vi "Vision Processing.vi"(4 "error in (no error)":errorcluster, 6 "CameraDevRef":T1) -> ()   [LabVIEW 2011]
uses:
  <vilib>/Rock Robotics/WPI/Camera/WPI_CameraDevRef.ctl
  Robot Global Data.vi
  <vilib>/vision/NI_Vision_Development_Module.lvlib
panel:
  in  "AntiDrift":dbl
  in  "Y AbsolVal Difference":dbl=0.25
  in  "Default Shooter Speed Dump":dbl=0.4
  in  "Scale":dbl=0.85
  in  "Minimum Power":dbl=0.22
  out "Aspect Ratio":dbl[](array[numeric])
  out "Offset":dbl
  out "Raw Turret":dbl
  out "Target X Coord":dbl
  out "Target Distance":dbl
  out "Distance Array":dbl[](array[numeric])
  in  "Dead Band":dbl=0.09
  out "Number of Rectangles Visible":dbl
  out "Y Position Array":dbl[](array[numeric])
  out "X Position Array":dbl[](array[numeric])
  in  "View":bool
  out "Target Info":T2(array[cluster])
  in  "Area Size Limit":i32=444
  in  "Particle Count Limit":i32=8
  in  "Score Limits":T3={"Rect Coverage"=76.0, "Aspect Ratio"=40.0, "X Edge Strength"=40.0, "Y Edge Strength"=60.0}
  in  "Processing":enum32{"Color", "Intensity", "Intensity Open"}(tab)=enum."Intensity"
  in  "Luminance":i32=255
  in  "Saturation":i32=255
  in  "Hue":i32(knob)=65 scale=0.0..255.0
  in  "Margins":cluster{"Hue":i32, "Sat":i32, "Lum":i32}={"Hue"=20, "Sat"=27, "Lum"=30} {"Sat" scale=0.0..40.0; "Lum" scale=0.0..40.0; "Hue" scale=0.0..40.0}
  in  "Range":cluster{"Lower value":sgl, "Upper value":sgl}={"Lower value"=151.52174, "Upper value"=255.0} {"Lower value" scale=0.0..255.0; "Upper value" scale=0.0..255.0}
  in  "Range":cluster{"Lower value":sgl, "Upper value":sgl}={"Lower value"=123.804344, "Upper value"=255.0} {"Lower value" scale=0.0..255.0; "Upper value" scale=0.0..255.0}
  in  "View":bool
  out "Processed Image":T4(plugin-control)
  out "Original Image":T4(plugin-control)
  # "Instructions:\nProcessing the reflective tape that is illuminated by a ring light can be based\non color or light intensity.\nParticles within the image are scored by rectangle coverage, aspect ratio, and\nfor being hollow with a bold edge. A particle is considered a target if all scores\nare above the score limits. Particles can be annotated -- surrounded by\na rectangle and scores drawn to the left .\nTo control the number of particles being scored, use the count limit and the size\nlimit."
  # "-0.065"
  # "(in)"
  # "To debug, Enable using the View button.\nFor color processing, you can click in the image to select the color for processing."
  # "Enable by clicking the View button.\nGreen scores are above the limit, orange are below. Inner/outer rect\nindicates all passed."
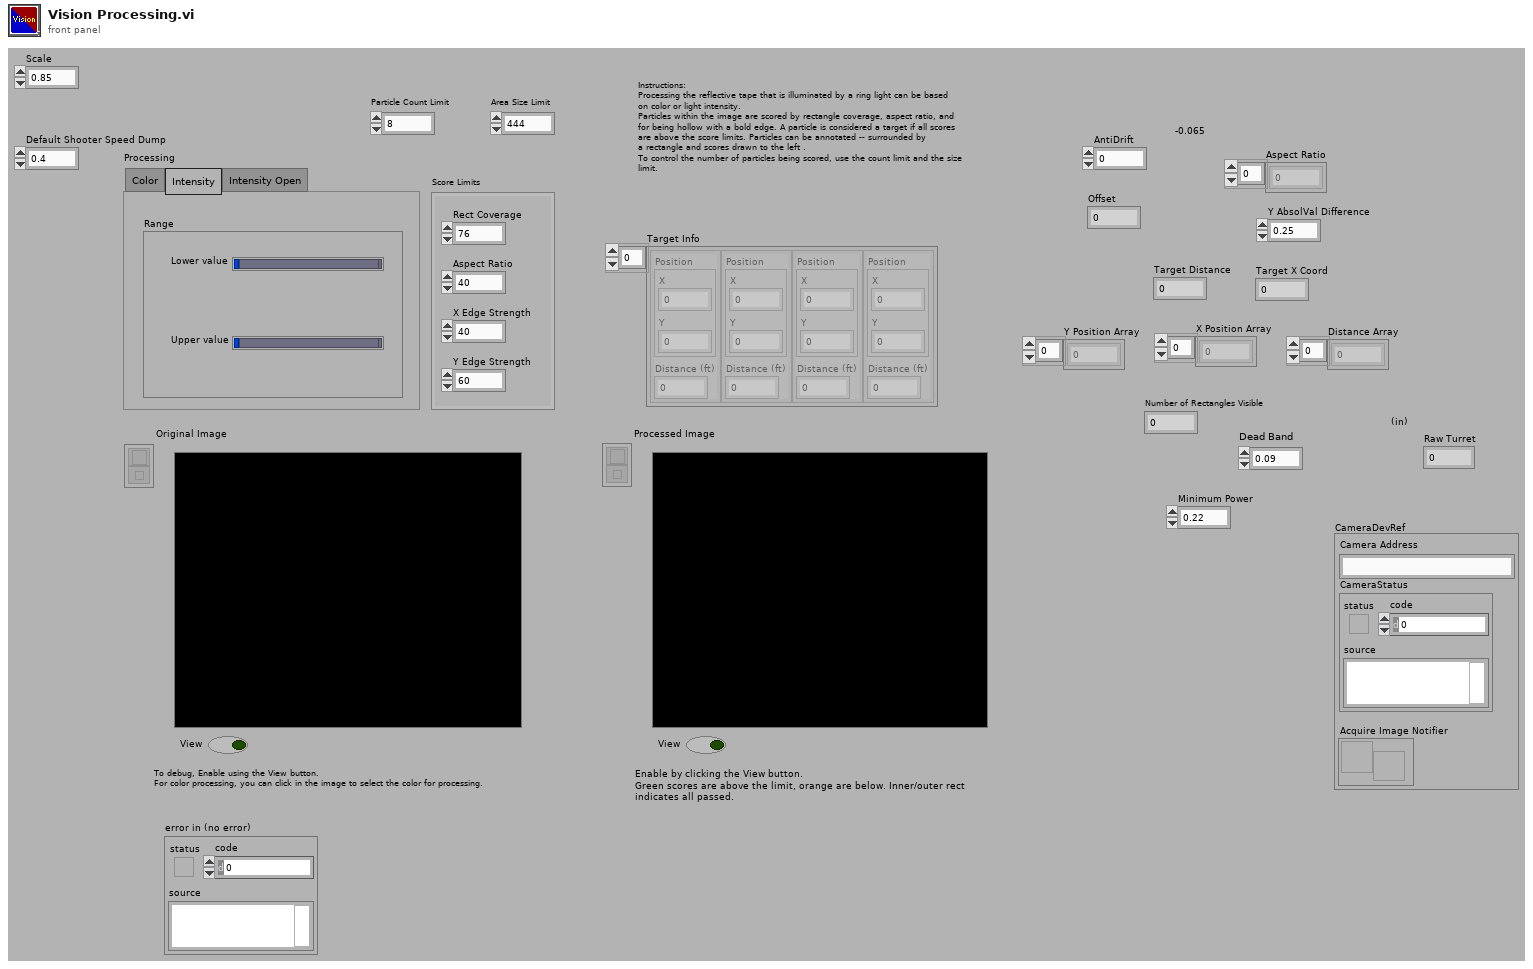
[diagram p1: front panel]
types:
  T1 = typedef "WPI_CameraDevRef.ctl" = cluster{"Camera Address":string, "CameraStatus":errorcluster, "Acquire Image Notifier":refnum<notifier>}
  T2 = cluster{"Position":cluster{"X":dbl, "Y":dbl}, "Distance (ft)":dbl}[]
  T3 = cluster{"Rect Coverage":dbl, "Aspect Ratio":dbl, "X Edge Strength":dbl, "Y Edge Strength":dbl}
  T4 = typedef "IMAQ Image.ctl" = refnum<image>
  T5 = typedef "Image Type" = u32
  T6 = enum32{"AutoM", "Close", "Dilate", "Erode", "Gradient", "Gradient out", "Gradient in", "Hit miss", "Open", "PClose", "POpen", "Thick", "Thin"}
  T7 = typedef "WPI_CameraImageSize.ctl" = enum16{"640x480", "320x240", "160x120"}
  T8 = cluster{"fps":i32, "compression":i32, "Image Size":T7}
  T9 = cluster{cluster{"Left":dbl, "Top":dbl, "Right":dbl, "Bottom":dbl}, dbl[]}[]
  T10 = cluster{"Left":dbl, "Top":dbl, "Right":dbl, "Bottom":dbl}
  T11 = cluster{"Target Center (-1 to 1)":cluster{"X":dbl, "Y":dbl}, "Distance (ft)":dbl}
  T12 = cluster{"Target Center (-1 to 1)":cluster{"X":dbl, "Y":dbl}, "Distance (ft)":dbl}[]
  T13 = typedef "WPI_JoystickDevRef.ctl" = cluster{"Device":T14}
  T14 = typedef "WPI_JoystickDeviceEnum.ctl" = enum16{"USB 1", "USB 2", "USB 3", "USB 4", "Kinect 1", "Kinect 2"}
  T15 = typedef "WPI_JoystickButtonState.ctl" = cluster{"Button 1":bool, "Button 2":bool, "Button 3":bool, "Button 4":bool, "Button 5":bool, "Button 6":bool, "Button 7":bool, "Button 8":bool, "Button 9":bool, "Button 10":bool, "Button 11":bool, "Button 12":bool}
  T16 = cluster{"axis 1 (x)":dbl, "axis 2 (y)":dbl, "axis 3 (throttle)":dbl, "axis 4":dbl, "axis 5":dbl, "axis 6":dbl}
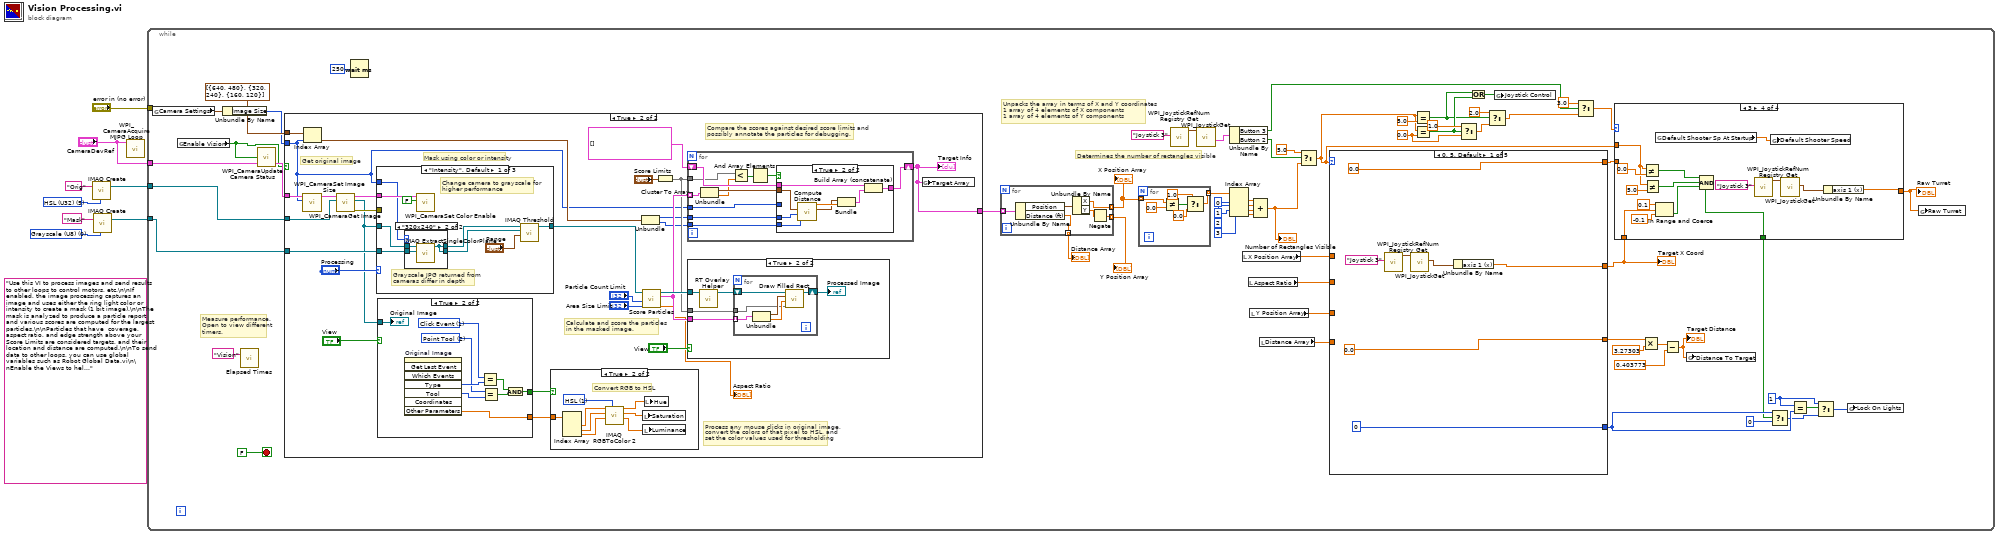
[diagram p0: block diagram]
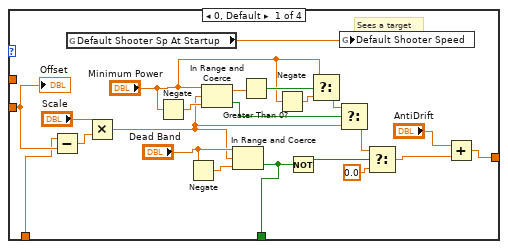
[diagram p2: hidden frame]
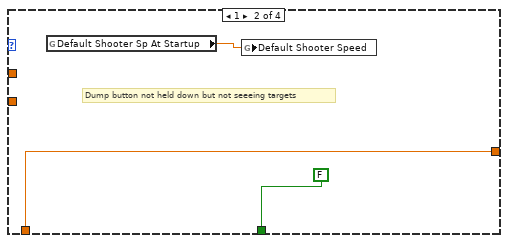
[diagram p3: hidden frame]
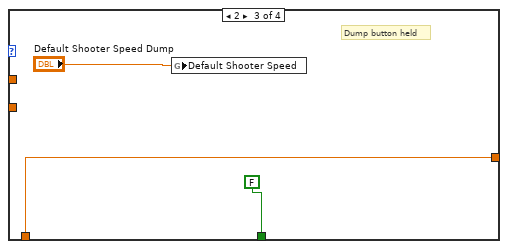
[diagram p4: hidden frame]
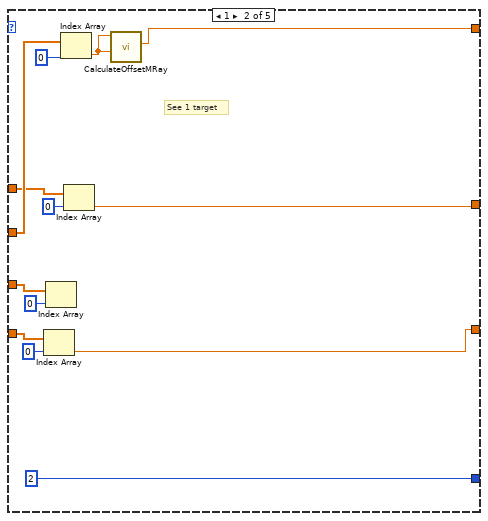
[diagram p5: hidden frame]
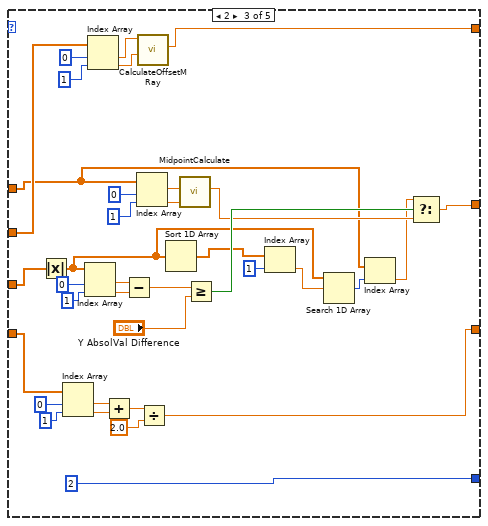
[diagram p6: hidden frame]
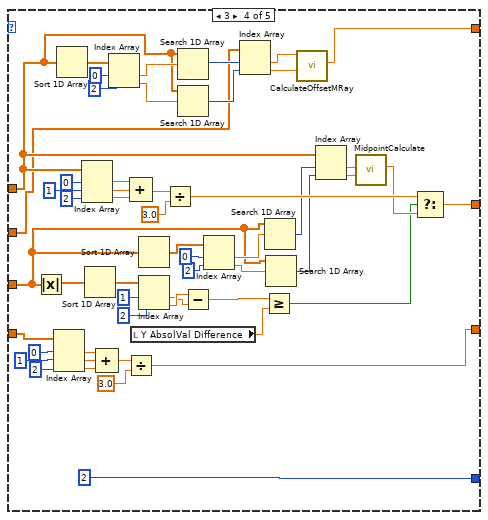
[diagram p7: hidden frame]
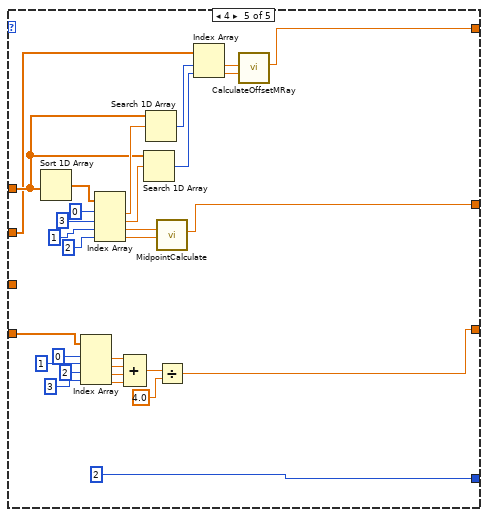
[diagram p8: hidden frame]
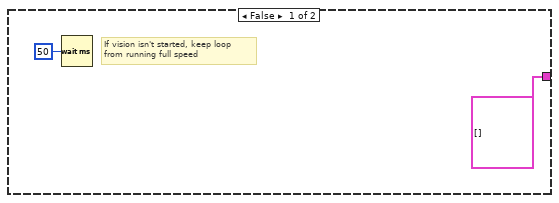
[diagram p9: hidden frame]
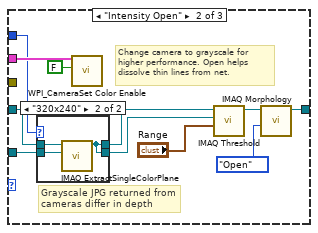
[diagram p12: hidden frame]
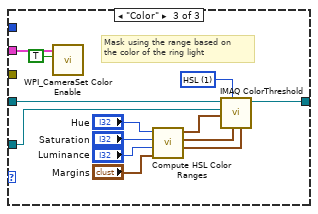
[diagram p14: hidden frame]
diagram:
  w3 = T5 0 items=["Grayscale (U8)", "Grayscale (I16)", "Grayscale (SGL)", "Complex (CSG)", "RGB (U32)", "HSL (U32)", "RGB (U64)", "Grayscale (U16)"] ("Image Type")
  (unwired) "Use this VI to process images and send results to other loops to control motors, etc.\n\nIf enabled, the image processing captures an image and uses either the ring light color or intensity to create a mask (1 bit image).\n\nThe mask is analyzed to produce a particle report and various scores are computed for the largest particles.\n\nParticles that have  coverage, aspect ratio, and edge strength above your Score Limits are considered targets, and their location and distance are computed.\n\nTo send data to other loops, you can use global variables such as Robot Global Data.vi\n\nEnable the Views to help debug color settings. Disable the View to speed up processing."
  w7 = T5 5 items=["Grayscale (U8)", "Grayscale (I16)", "Grayscale (SGL)", "Complex (CSG)", "RGB (U32)", "HSL (U32)", "RGB (U64)", "Grayscale (U16)"] ("Image Type")
  n1 = call "IMAQ Create"("Image Name"="Orig", "Image Type"=w7) -> ("New Image"=w6:T4)  [unwired: 2 in, 2 out]
  n2 = call "IMAQ Create"("Image Name"="Mask", "Image Type"=w3) -> ("New Image"=w1:T4)  [unwired: 2 in, 2 out]
  n3 = call <vilib>:"WPI_CameraAcquire MJPG Loop.vi"("CameraDevRef"="CameraDevRef") -> ()  [unwired: 11 in]
  n4 = while {
    tunnel: w6 -> [w69]
    tunnel: "CameraDevRef" -> [w68]
    tunnel: "error in (no error)" -> [_]
    tunnel: w1 -> [w64]
    stop <- FALSE stop-if-true
    w17 = 0.0 ("y")
    w34 = 1 ("y")
    # "Determines the number of rectangles visible"
    # "Unpacks the array in terms of X and Y coordinates\n1 array of 4 elements of X components\n1 array of 4 elements of Y components"
    # "Measure performance.\nOpen to view different\ntimers."
    n5 = global read "Robot Global Data.vi" "Camera Settings"() -> (w62:T8)
    n6 = global read "Robot Global Data.vi" "Enable Vision"() -> (w66:bool)
    n7 = Unbundle By Name(w62) -> ("Image Size"=w61:T7)
    n8 = call "Elapsed Times.vi"("Call Name"="Vision") -> ()  [unwired: 2 in, 1 out]
    n9 = call <vilib>:"WPI_CameraUpdate Camera Status.vi"("CameraDevRef In"=w68, "Enable Vision"=w66) -> ("CameraDevRef Out"=w67:T1)  [unwired: 3 in]
    n10 = case shown="True" w66 {
      tunnel: w69 -> [_ w284]
      tunnel: w67 -> [_ w280]
      tunnel: w64 -> [_ w271]
      tunnel: cluster{i32, i32}[] [{640, 480}, {320, 240}, {160, 120}] -> [_ w275]
      tunnel: w61 -> [_ w268]
      tunnel: [T2 [] w269] -> w60
      frame False {
        # "If vision isn't started, keep loop\nfrom running full speed"
        n11 = Wait (ms)(milliseconds to wait=u32 50) -> ()  [unwired: 1 out]
      }
      frame True {
        # "Compare the scores against desired score limits and\npossibly annotate the particles for debugging."
        # "Process any mouse clicks in original image,\nconvert the colors of that pixel to HSL, and\nset the color values used for thresholding"
        # "Calculate and score the particles\nin the masked image."
        # "Mask using color or intensity"
        # "Get original image"
        n12 = call <vilib>:"WPI_CameraSet Image Size.vi"("Image Size"=w268, "CameraDevRef"=w280) -> ("CameraDevRef Out"=w281:T1)  [unwired: 8 in, 1 out]
        n13 = Index Array(array=w275, index=w268) -> (element=w272:cluster{i32, i32})
        n14 = call <vilib>:"WPI_CameraGet Image.vi"("Image"=w284, "CameraDevRef"=w281) -> ("error out"=w282:errorcluster, "Image Out"=w270:T4, "CameraDevRef Out"=w283:T1)  [unwired: 7 in]
        n15 = case shown="\"Intensity\", Default" "Processing" {
          tunnel: w270 -> [w306 w318 w344]
          tunnel: [w309 w323 w343] -> w278
          tunnel: w283 -> [w307 w321 w334]
          tunnel: w282 -> [_ _ _]
          tunnel: w271 -> [w305 w319 w332]
          tunnel: w268 -> [w304 w320 _]
          frame "Intensity", Default {
            # "Grayscale JPG returned from\ncameras differ in depth"
            # "Change camera to grayscale for\nhigher performance"
            n16 = case shown="\"320x240\"" w304 {
              tunnel: w306 -> [w312 w315]
              tunnel: w305 -> [w311 w314]
              tunnel: [w312 w313] -> w303
              tunnel: [w311 w313] -> w302
              frame "640x480", Default {
              }
              frame "320x240" {
                n17 = call "IMAQ ExtractSingleColorPlane"("Image Dst"=w314, "Image Src"=w315) -> ("Image Dst Out"=w313:T4)  [unwired: 8 in, 1 out]
              }
            }
            n18 = call <vilib>:"WPI_CameraSet Color Enable.vi"("Color Enabled"=FALSE, "CameraDevRef"=w307) -> ()  [unwired: 8 in, 2 out]
            n19 = call "IMAQ Threshold"("Range"="Range", "Image Dst"=w302, "Image Src"=w303) -> ("Image Dst Out"=w309:T4)  [unwired: 3 in, 5 out]
          }
          frame "Intensity Open" {
            # "Grayscale JPG returned from\ncameras differ in depth"
            # "Change camera to grayscale for\nhigher performance. Open helps\ndissolve thin lines from net."
            n20 = case shown="\"320x240\"" w320 {
              tunnel: w318 -> [w328 w331]
              tunnel: w319 -> [w327 w330]
              tunnel: [w328 w329] -> w317
              tunnel: [w327 w329] -> w316
              frame "640x480", Default {
              }
              frame "320x240" {
                n21 = call "IMAQ ExtractSingleColorPlane"("Image Dst"=w330, "Image Src"=w331) -> ("Image Dst Out"=w329:T4)  [unwired: 8 in, 1 out]
              }
            }
            n22 = call <vilib>:"WPI_CameraSet Color Enable.vi"("Color Enabled"=FALSE, "CameraDevRef"=w321) -> ()  [unwired: 8 in, 2 out]
            n23 = call "IMAQ Threshold"("Range"="Range", "Image Dst"=w316, "Image Src"=w317) -> ("Image Dst Out"=w324:T4)  [unwired: 3 in, 5 out]
            n24 = call "IMAQ Morphology"("Operation"=T6."Open", "Image Src"=w324) -> ("Image Dst Out"=w323:T4)  [unwired: 8 in, 1 out]
          }
          frame "Color" {
            w342 = u16 1 items=["RGB", "HSL", "HSV", "HSI"] ("Color Mode")
            # "Mask using the range based on\nthe color of the ring light"
            n25 = call <vilib>:"WPI_CameraSet Color Enable.vi"("Color Enabled"=TRUE, "CameraDevRef"=w334) -> ()  [unwired: 8 in, 2 out]
            n26 = call "Compute HSL Color Ranges.vi"("Margins"="Margins", "Luminance"="Luminance", "Saturation"="Saturation", "Hue"="Hue") -> ("Lum Range"=w339:cluster{i32, i32}, "Sat Range"=w340:cluster{i32, i32}, "Hue Range"=w341:cluster{i32, i32})  [unwired: 5 in]
            n27 = call "IMAQ ColorThreshold"("Blue or Luma or Val or Inten Range"=w339, "Green or Sat Range"=w340, "Color Mode"=w342, "Red or Hue Range"=w341, "Image Dst"=w332, "Image Src"=w344) -> ("Image Dst Out"=w343:T4)  [unwired: 4 in, 1 out]
          }
        }
        n28 = case shown="True" "View" {
          tunnel: w270 -> [_ w364]
          tunnel: [_ w359] -> w277
          tunnel: [_ w356] -> w276
          frame False {
          }
          frame True {
            w357 = 2 items=["None", "Selection Tool", "Point Tool", "Line Tool", "Rectangle Tool", "Oval Tool", "Polygon Tool", "ClosedFreehandTool", "Annulus Tool", "Rotated Rectangle Tool", "Zoom Tool", "Pan Tool", "Polyline Tool", "Freehand Tool"] ("Tool")
            w358 = 1 items=["No Event"=0, "Click Event"=1, "Draw Event"=2, "Size Event"=4, "Scroll Event"=5, "Double Click Event"=8] ("Type")
            n29 = invoke on="Original Image" class="ImageControl" method="Get Last Event"() -> ("Type"=w360:i32, "Tool"=w363:i32, "Other Parameters"=w356:sgl[])  [unwired: 8 in, 5 out]
            n30 = Equal?(x=w358, y=w360) -> (x = y?=w361:bool)
            n31 = Equal?(x=w357, y=w363) -> (x = y?=w362:bool)
            n32 = And(x=w361, y=w362) -> (x .and. y?=w359:bool)
            "Original Image" <- w364
          }
        }
        n33 = case shown="True" w277 {
          tunnel: w276 -> [_ w301]
          frame False {
          }
          frame True {
            w300 = u16 1 items=["RGB", "HSL", "HSV", "HSI", "CIE L*a*b*", "CIE XYZ"] ("Color Mode")
            # "Convert RGB to HSL"
            n34 = Index Array(array=w301) -> (element #1=w299:sgl, element #2=w297:sgl, element #3=w295:sgl)  [unwired: 3 in]
            n35 = call "IMAQ RGBToColor 2"("Color Mode"=w300, "Blue value"=w295, "Green value"=w297, "Red value"=w299) -> ("Blue or Luma or Val or Inten or Z or b*value"=w294:dbl, "Green or Sat or Y or a* value"=w296:dbl, "Red or Hue or X or L* value"=w298:dbl)  [unwired: 4 in, 1 out]
            n36 = local write "Saturation"(w296) -> ()
            n37 = local write "Luminance"(w294) -> ()
            n38 = local write "Hue"(w298) -> ()
          }
        }
        n39 = Unbundle(w272) -> (w274:i32, w273:i32)
        n40 = call "Score Particles.vi"("Area Size Limit"="Area Size Limit", "Particle Count Limit"="Particle Count Limit", "Image Refnum in"=w278) -> ("Aspect Ratio"=→"Aspect Ratio":dbl[], "Scored Particle Info"=w289:T9, "Image Refnum out"=w292:T4)  [unwired: 6 in]
        n41 = Cluster To Array(cluster="Score Limits") -> (array=w287:dbl[])
        n42 = for {
          shift-right: [w374] -> w269
          shift-left: T2 [] -> [w375]
          tunnel: w274 -> [w373]
          tunnel: w289 -> [w371] mode=indexing
          tunnel: w287 -> [w366]
          tunnel: w268 -> [w370]
          tunnel: w273 -> [w365]
          n43 = Unbundle(w371) -> (w372:T10, w367:dbl[])
          n44 = Less?(x=w366, y=w367) -> (x < y?=w369:bool[])
          n45 = And Array Elements(Boolean array=w369) -> (logical AND=w368:bool)
          n46 = case shown="True" w368 {
            tunnel: w375 -> [w376 w384]
            tunnel: [w376 w383] -> w374
            tunnel: w372 -> [_ w379]
            tunnel: w373 -> [_ w381]
            tunnel: w370 -> [_ _]
            tunnel: w365 -> [_ w378]
            frame False {
            }
            frame True {
              n47 = call "Compute Distance.vi"("Y Image Resolution"=w378, "X Image Resolution"=w381, "Bounding Box"=w379) -> ("Target Center (-1 to 1)"=w377:cluster{"X":dbl, "Y":dbl}, "Distance (ft)"=w380:dbl)  [unwired: 7 in]
              n48 = Bundle("Target Center (-1 to 1)"=w377, "Distance (ft)"=w380) -> (w382:T11)  [unwired: 1 in]
              n49 = Build Array (concatenate)(w384, w382) -> (w383:T12)
            }
          }
        }
        "Target Info" <- w269
        n50 = case shown="True" "View" {
          tunnel: w292 -> [_ w346]
          tunnel: w289 -> [_ w348]
          tunnel: w287 -> [_ w347]
          frame False {
          }
          frame True {
            n51 = call "RT Overlay Helper.vi"("Refnum in"=w346) -> ("Refnum out"=w349:T4)  [unwired: 10 in]
            n52 = for {
              shift-right: [w354] -> w345
              shift-left: w349 -> [w355]
              tunnel: w348 -> [w351] mode=indexing
              tunnel: w347 -> [w350]
              n53 = Unbundle(w351) -> (w352:T10, w353:dbl[])
              n54 = call "Draw Filled Rect.vi"("Limits"=w350, "Scores"=w353, "Bounding Box"=w352, "image in"=w355) -> ("image out"=w354:T4)  [unwired: 7 in]
            }
            "Processed Image" <- w345
          }
        }
        n55 = global write "Robot Global Data.vi" "Target Array"(w269) -> ()
      }
    }
    n56 = Wait (ms)(milliseconds to wait=u32 250) -> ()  [unwired: 1 out]
    n57 = for {
      tunnel: [w262] -> w40 mode=indexing
      tunnel: [w263] -> w50 mode=indexing
      tunnel: w60 -> [w260] mode=indexing
      tunnel: [w259] -> w52 mode=indexing
      n58 = Unbundle By Name(w260) -> ("Position"=w264:cluster{"X":dbl, "Y":dbl}, "Distance (ft)"=w259:dbl)
      n59 = Unbundle By Name(w264) -> ("X"=w263:dbl, "Y"=w261:dbl)
      n60 = Negate(x=w261) -> (-x=w262:dbl)
    }
    "X Position Array" <- w50
    "Y Position Array" <- w40
    "Distance Array" <- w52
    n61 = for {
      tunnel: w50 -> [w118] mode=indexing
      tunnel: [w114] -> w49 mode=indexing
      n62 = Not Equal?(x=w118, y=0.0) -> (x != y?=w117:bool)
      n63 = Select(t=1.0, s=w117, f=0.0) -> (s? t:f=w114:dbl)
    }
    n64 = call <vilib>:"WPI_JoystickRefNum Registry Get.vi"("refnum name"="Joystick 3") -> ("JoystickDevRef"=w39:T13)  [unwired: 9 in, 1 out]
    n65 = call <vilib>:"WPI_JoystickGet.vi"("JoystickDevRef"=w39) -> ("Buttons"=w37:T15)  [unwired: 4 in, 2 out]
    n66 = Unbundle By Name(w37) -> ("Button 3"=w11:bool, "Button 2"=w36:bool)
    n67 = Index Array(array=w49, index #1=0 ("index"), index #2=1 ("index"), index #3=2 ("index"), index #4=3 ("index")) -> (element #1=w47:dbl, element #2=w48:dbl, element #3=w46:dbl, element #4=w45:dbl)
    n68 = local read "X Position Array"() -> (w51:dbl[])
    n69 = local read "Aspect Ratio"() -> (w29:dbl[])
    n70 = local read "Y Position Array"() -> (w53:dbl[])
    n71 = Compound Arithmetic op=ADD(w47, w48, w46, w45) -> (w30:dbl)
    "Number of Rectangles Visible" <- w30
    n72 = local read "Distance Array"() -> (w54:dbl[])
    n73 = Select(t=5.0, s=w36, f=w30) -> (s? t:f=w9:dbl)
    n74 = case shown="0, 5, Default" w9 {
      tunnel: w51 -> [_ w134 w141 w183 w234]
      tunnel: [w122 w133 w165 w217 w257] -> w27
      tunnel: w53 -> [_ w131 w164 w195 _]
      tunnel: w54 -> [_ w129 w153 w226 w254]
      tunnel: [0 2 2 2 2] -> w33
      tunnel: [0.0 ("Offset") w136 w170 w176 w243] -> w28
      tunnel: w29 -> [_ w139 w173 w179 w229]
      tunnel: [0.0 w128 w148 w219 w244] -> w22
      frame 0, 5, Default {
        n75 = call <vilib>:"WPI_JoystickRefNum Registry Get.vi"("refnum name"="Joystick 3") -> ("JoystickDevRef"=w121:T13)  [unwired: 9 in, 1 out]
        n76 = call <vilib>:"WPI_JoystickGet.vi"("JoystickDevRef"=w121) -> ("Axes"=w123:T16)  [unwired: 4 in, 2 out]
        n77 = Unbundle By Name(w123) -> ("axis 1 (x)"=w122:dbl)
      }
      frame 1 {
        # "See 1 target"
        n78 = Index Array(array=w129, index=0) -> (element=w128:dbl)
        n79 = Index Array(array=w131, index=0) -> ()  [unwired: 1 out]
        n80 = Index Array(array=w139, index=0) -> (element=w137:dbl)
        n81 = Index Array(array=w134, index=0) -> (element=w133:dbl)
        n82 = call "CalculateOffsetMRay.vi"("AR2"=w137, "AR1"=w137) -> ("Offset"=w136:dbl)  [unwired: 9 in]
      }
      frame 2 {
        n83 = Absolute Value(x=w164) -> (abs(x)=w144:dbl[])
        n84 = Index Array(array=w153, index #1=0 ("index"), index #2=1 ("index")) -> (element #1=w151:dbl, element #2=w152:dbl)
        n85 = Index Array(array=w144, index #1=0 ("index"), index #2=1 ("index")) -> (element #1=w160:dbl, element #2=w161:dbl)
        n86 = Index Array(array=w173, index #1=0 ("index"), index #2=1 ("index")) -> (element #1=w172:dbl, element #2=w171:dbl)
        n87 = Add(x=w151, y=w152) -> (x+y=w150:dbl)
        n88 = Subtract(x=w160, y=w161) -> (x-y=w159:dbl)
        n89 = Index Array(array=w141, index #1=0 ("index"), index #2=1 ("index")) -> (element #1=w166:dbl, element #2=w167:dbl)
        n90 = call "CalculateOffsetMRay.vi"("AR2"=w171, "AR1"=w172) -> ("Offset"=w170:dbl)  [unwired: 9 in]
        n91 = Divide(x=w150, y=2.0) -> (x/y=w148:dbl)
        n92 = Sort 1D Array(array=w144) -> (sorted array=w146:dbl[])
        n93 = call "MidpointCalculate.vi"("X2"=w167, "X1"=w166) -> ("Midpoint"=w156:dbl)  [unwired: 9 in]
        n94 = Greater Or Equal?(x=w159, y="Y AbsolVal Difference") -> (x >= y?=w157:bool)
        n95 = Index Array(array=w146, index=1) -> (element=w143:dbl)
        n96 = Search 1D Array(1D array=w144, element=w143) -> (index of element=w142:i32)  [unwired: 1 in]
        n97 = Index Array(array=w141, index=w142) -> (element=w140:dbl)
        n98 = Select(t=w140, s=w157, f=w156) -> (s? t:f=w165:dbl)
      }
      frame 3 {
        n99 = Absolute Value(x=w195) -> (abs(x)=w216:dbl[])
        n100 = Index Array(array=w226, index #1=0 ("index"), index #2=1 ("index"), index #3=2 ("index")) -> (element #1=w222:dbl, element #2=w223:dbl, element #3=w224:dbl)
        n101 = Sort 1D Array(array=w183) -> (sorted array=w187:dbl[])
        n102 = Index Array(array=w183, index #1=0 ("index"), index #2=1 ("index"), index #3=2 ("index")) -> (element #1=w204:dbl, element #2=w206:dbl, element #3=w205:dbl)
        n103 = Sort 1D Array(array=w216) -> (sorted array=w200:dbl[])
        n104 = Compound Arithmetic op=ADD(w222, w223, w224) -> (w221:dbl)
        n105 = Index Array(array=w187, index #1=0 ("index"), index #2=2 ("index")) -> (element #1=w184:dbl, element #2=w182:dbl)
        n106 = Divide(x=w221, y=3.0) -> (x/y=w219:dbl)
        n107 = Compound Arithmetic op=ADD(w204, w206, w205) -> (w203:dbl)
        n108 = local read "Y AbsolVal Difference"() -> (w210:dbl)
        n109 = Sort 1D Array(array=w195) -> (sorted array=w199:dbl[])
        n110 = Index Array(array=w200, index #1=1 ("index"), index #2=2 ("index")) -> (element #1=w212:dbl, element #2=w213:dbl)
        n111 = Divide(x=w203, y=3.0) -> (x/y=w201:dbl)
        n112 = Search 1D Array(1D array=w183, element=w184) -> (index of element=w181:i32)  [unwired: 1 in]
        n113 = Search 1D Array(1D array=w183, element=w182) -> (index of element=w180:i32)  [unwired: 1 in]
        n114 = Subtract(x=w213, y=w212) -> (x-y=w211:dbl)
        n115 = Index Array(array=w199, index #1=0 ("index"), index #2=2 ("index")) -> (element #1=w196:dbl, element #2=w194:dbl)
        n116 = Index Array(array=w179, index #1=w181, index #2=w180) -> (element #1=w178:dbl, element #2=w177:dbl)
        n117 = Greater Or Equal?(x=w211, y=w210) -> (x >= y?=w188:bool)
        n118 = Search 1D Array(1D array=w195, element=w196) -> (index of element=w193:i32)  [unwired: 1 in]
        n119 = Search 1D Array(1D array=w195, element=w194) -> (index of element=w192:i32)  [unwired: 1 in]
        n120 = call "CalculateOffsetMRay.vi"("AR2"=w177, "AR1"=w178) -> ("Offset"=w176:dbl)  [unwired: 9 in]
        n121 = Index Array(array=w183, index #1=w193, index #2=w192) -> (element #1=w190:dbl, element #2=w191:dbl)
        n122 = call "MidpointCalculate.vi"("X2"=w191, "X1"=w190) -> ("Midpoint"=w189:dbl)  [unwired: 9 in]
        n123 = Select(t=w201, s=w188, f=w189) -> (s? t:f=w217:dbl)
      }
      frame 4 {
        n124 = Sort 1D Array(array=w234) -> (sorted array=w258:dbl[])
        n125 = Index Array(array=w254, index #1=0 ("index"), index #2=1 ("index"), index #3=2 ("index"), index #4=3 ("index")) -> (element #1=w251:dbl, element #2=w250:dbl, element #3=w249:dbl, element #4=w248:dbl)
        n126 = Index Array(array=w258, index #1=0 ("index"), index #2=3 ("index"), index #3=1 ("index"), index #4=2 ("index")) -> (element #1=w235:dbl, element #2=w236:dbl, element #3=w242:dbl, element #4=w241:dbl)
        n127 = Compound Arithmetic op=ADD(w251, w250, w249, w248) -> (w247:dbl)
        n128 = Search 1D Array(1D array=w234, element=w236) -> (index of element=w231:i32)  [unwired: 1 in]
        n129 = Search 1D Array(1D array=w234, element=w235) -> (index of element=w230:i32)  [unwired: 1 in]
        n130 = call "MidpointCalculate.vi"("X2"=w241, "X1"=w242) -> ("Midpoint"=w257:dbl)  [unwired: 9 in]
        n131 = Divide(x=w247, y=4.0) -> (x/y=w244:dbl)
        n132 = Index Array(array=w229, index #1=w230, index #2=w231) -> (element #1=w233:dbl, element #2=w232:dbl)
        n133 = call "CalculateOffsetMRay.vi"("AR2"=w232, "AR1"=w233) -> ("Offset"=w243:dbl)  [unwired: 9 in]
      }
    }
    "Target X Coord" <- w27
    n134 = Equal?(x=w9, y=5.0) -> (x = y?=w15:bool)
    n135 = Equal?(x=w9, y=w17) -> (x = y?=w16:bool)
    n136 = Select(t=1.0, s=w16, f=w17) -> (s? t:f=w20:dbl)
    n137 = Or(x=w15, y=w16) -> (x .or. y?=w14:bool)
    n138 = Select(t=2.0, s=w15, f=w20) -> (s? t:f=w13:dbl)
    n139 = global write "Robot Global Data.vi" "Joystick Control"(w14) -> ()
    n140 = Select(t=3.0, s=w11, f=w13) -> (s? t:f=w12:dbl)
    n141 = case shown="3" w12 {
      tunnel: w28 -> [w91 _ _ _]
      tunnel: w27 -> [w90 w95 w98 w102]
      tunnel: [w73 w95 w98 w109] -> w58
      tunnel: [w76 FALSE FALSE w104] -> w26
      tunnel: w9 -> [_ _ _ w103]
      frame 0, Default {
        # "Sees a target"
        n142 = Subtract(x=w90, y=w91) -> (x-y=w88:dbl)
        n143 = global read "Robot Global Data.vi" "Default Shooter Sp At Startup"() -> (w71:dbl)
        n144 = Multiply(x="Scale", y=w88) -> (x*y=w79:dbl)
        n145 = Negate(x="Minimum Power") -> (-x=w86:dbl)
        n146 = Negate(x="Dead Band") -> (-x=w92:dbl)
        n147 = In Range and Coerce(upper limit="Minimum Power", x=w79, lower limit=w86) -> (coerced(x)=w82:dbl, In Range?=w83:bool)
        n148 = In Range and Coerce(upper limit="Dead Band", x=w79, lower limit=w92) -> (In Range?=w76:bool)  [unwired: 1 out]
        n149 = Greater Than 0?(x=w82) -> (x > 0?=w81:bool)
        n150 = Negate(x="Minimum Power") -> (-x=w78:dbl)
        n151 = Not(x=w76) -> (.not. x?=w77:bool)
        n152 = Select(t="Minimum Power", s=w81, f=w78) -> (s? t:f=w80:dbl)
        n153 = Select(t=w80, s=w83, f=w79) -> (s? t:f=w84:dbl)
        n154 = global write "Robot Global Data.vi" "Default Shooter Speed"(w71) -> ()
        n155 = Select(t=w84, s=w77, f=0.0) -> (s? t:f=w74:dbl)
        n156 = Add(x="AntiDrift", y=w74) -> (x+y=w73:dbl)
        "Offset" <- w91
      }
      frame 1 {
        # "Dump button not held down but not seeeing targets"
        n157 = global read "Robot Global Data.vi" "Default Shooter Sp At Startup"() -> (w93:dbl)
        n158 = global write "Robot Global Data.vi" "Default Shooter Speed"(w93) -> ()
      }
      frame 2 {
        # "Dump button held"
        n159 = global write "Robot Global Data.vi" "Default Shooter Speed"("Default Shooter Speed Dump") -> ()
      }
      frame 3 {
        n160 = Not Equal?(x=w103, y=0.0) -> (x != y?=w105:bool)
        n161 = Not Equal?(x=w103, y=5.0) -> (x != y?=w106:bool)
        n162 = In Range and Coerce(upper limit=0.1, x=w102, lower limit=-0.1) -> (In Range?=w100:bool)  [unwired: 1 out]
        n163 = global read "Robot Global Data.vi" "Default Shooter Sp At Startup"() -> (w113:dbl)
        n164 = Compound Arithmetic op=AND(w105, w106, w100) -> (w104:bool)
        n165 = call <vilib>:"WPI_JoystickRefNum Registry Get.vi"("refnum name"="Joystick 3") -> ("JoystickDevRef"=w112:T13)  [unwired: 9 in, 1 out]
        n166 = global write "Robot Global Data.vi" "Default Shooter Speed"(w113) -> ()
        n167 = call <vilib>:"WPI_JoystickGet.vi"("JoystickDevRef"=w112) -> ("Axes"=w111:T16)  [unwired: 4 in, 2 out]
        n168 = Unbundle By Name(w111) -> ("axis 1 (x)"=w109:dbl)
      }
    }
    "Raw Turret" <- w58
    n169 = Multiply(x=w22, y=3.27303) -> (x*y=w25:dbl)
    n170 = Subtract(x=w25, y=0.403773) -> (x-y=w56:dbl)
    "Target Distance" <- w56
    n171 = global write "Robot Global Data.vi" "Distance To Target"(w56) -> ()
    n172 = Select(t=w33, s=w26, f=0) -> (s? t:f=w31:i32)
    n173 = Equal?(x=w34, y=w33) -> (x = y?=w35:bool)
    n174 = Select(t=w34, s=w35, f=w31) -> (s? t:f=w57:i32)
    n175 = global write "Robot Global Data.vi" "Lock On Lights"(w57) -> ()
    n176 = global write "Robot Global Data.vi" "Raw Turret"(w58) -> ()
  }
